vi "WAV_Save.vi"(10 "file string":string, 11 "file (use dialog)":path) -> (0 "error out":errorcluster, 3 "File Size":i32)   [LabVIEW 2022 SP3]
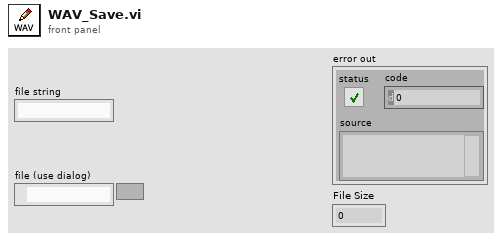
[diagram p1: front panel]
types:
  T1 = enum16{"big-endian, network order", "native, host order", "little-endian"}
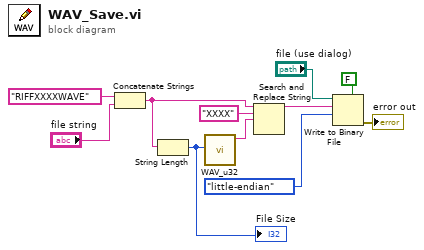
[diagram p0: block diagram]
diagram:
  n1 = Concatenate Strings("RIFFXXXXWAVE" ("string"), "file string") -> (w8:string)
  n2 = String Length(string=w8) -> (length=w6:i32)
  "File Size" <- w6
  n3 = call "WAV_u32.vi"("u32"=w6) -> ("String out"=w5:string)  [unwired: 10 in]
  n4 = Search and Replace String(input string=w8, search string="XXXX", replace string=w5) -> (result string=w11:string)  [unwired: 5 in, 3 out]
  n5 = Write to Binary File(file (use dialog)="file (use dialog)", data=w11, 5:FALSE ("prepend array or string size? (T)"), 9:T1."little-endian" ("byte order (0:big-endian, network order)")) -> (error out=→"error out":errorcluster)  [unwired: 2 in, 2 out]
